vi "HEWH Flow Adjustment.vi"(0 "VISA session":refnum<visa-resource-name>="MW100", 1 "Configuration":T1=enum."SRK500,Station1,5GPM FR", 2 "Semiphore":T2, 5 "GPM Target(3)":dbl=3.0, 7 "GPM reading":dbl, 9 "Flow rate setting In":dbl=2.9360496277915633, 11 "Error In":errorcluster, 12 "Elapsed Time (sec)":dbl format="%.2f", 13 "Flow Adjust Time (3s)":dbl=3.0, 14 "K(0.1)":dbl=0.1) -> (4 "VISA session out":refnum<visa-resource-name>, 6 "Flow rate setting Out":dbl, 15 "Error Out":errorcluster)   [LabVIEW 2012]
uses:
  TestedFlowratesScenarios.ctl
  Intellifaucet/Intellfaucet Mode.ctl
panel:
  in  "ErrorPassBand(%)":dbl=0.05
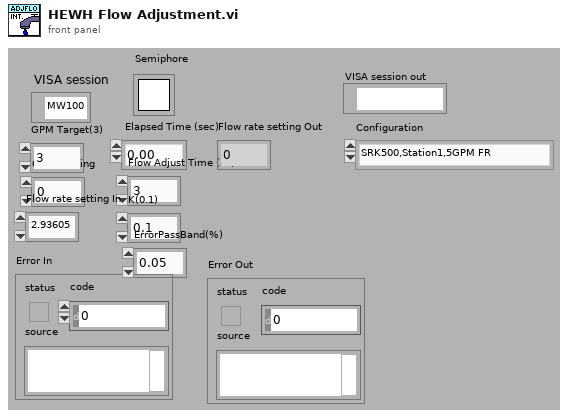
[diagram p1: front panel]
types:
  T1 = typedef "TestedFlowratesScenarios.ctl" = enum16{"DRK500,Station1", "DRK375,Lab", "SRK500,Station1,5GPM FR", "DRK375,STATION3,1/2\"HOSE", "DRK500,Station1,downspout", "DRK375,Station3,thruEcocute", "DRK375,Station3,purge", "Build2,2B,Purge", "Global, Purge", "Global, Tank"}
  T2 = typedef "Semaphore RefNum" = refnum<k1>
  T3 = typedef "Intellfaucet Mode.ctl" = enum16{"Adjust Temp", "Adjust Flow", "Start Flow", "Stop Flow"}
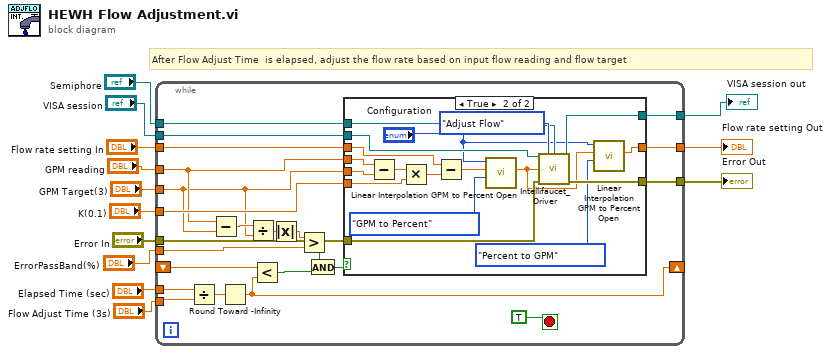
[diagram p0: block diagram]
diagram:
  # "After Flow Adjust Time  is elapsed, adjust the flow rate based on input flow reading and flow target"
  n1 = while {
    tunnel: "Elapsed Time (sec)" -> [w35]
    tunnel: "Flow Adjust Time (3s)" -> [w34]
    shift-right: [w24] -> _
    shift-left: _ -> [w25]
    tunnel: "VISA session" -> [w32]
    tunnel: "Semiphore" -> [w31]
    tunnel: "Error In" -> [w30]
    tunnel: [w29] -> w8
    tunnel: "GPM reading" -> [w20]
    tunnel: "GPM Target(3)" -> [w18]
    tunnel: "K(0.1)" -> [w28]
    tunnel: "Flow rate setting In" -> [w27]
    tunnel: [w26] -> w3
    tunnel: [w23] -> w2
    tunnel: "ErrorPassBand(%)" -> [w17]
    stop <- TRUE stop-if-true
    n2 = Divide(x=w35, y=w34) -> (x/y=w33:dbl)
    n3 = Subtract(x=w20, y=w18) -> (x-y=w19:dbl)
    n4 = Round Toward -Infinity(1:w33) -> (0:w24:dbl)
    n5 = Divide(x=w19, y=w18) -> (x/y=w14:dbl)
    n6 = Less?(x=w25, y=w24) -> (x < y?=w22:bool)
    n7 = Absolute Value(x=w14) -> (abs(x)=w15:dbl)
    n8 = Greater?(x=w15, y=w17) -> (0:w16:bool)
    n9 = And(x=w16, y=w22) -> (x .and. y?=w21:bool)
    n10 = case shown="True" w21 {
      tunnel: w32 -> [w37 w56]
      tunnel: w31 -> [_ w55]
      tunnel: w30 -> [w39 w54]
      tunnel: [w39 w53] -> w29
      tunnel: w28 -> [_ w51]
      tunnel: w18 -> [_ w50]
      tunnel: w20 -> [_ w49]
      tunnel: w27 -> [w38 w47]
      tunnel: [w38 w43] -> w26
      tunnel: [w37 w45] -> w23
      frame False {
      }
      frame True {
        n11 = Subtract(x=w49, y=w50) -> (x-y=w52:dbl)
        n12 = Multiply(x=w52, y=w51) -> (x*y=w48:dbl)
        n13 = Subtract(x=w47, y=w48) -> (x-y=w46:dbl)
        n14 = call "Linear Interpolation GPM to Percent Open.vi"("Interp Direction"=enum16{"GPM to Percent", "Percent to GPM"}."GPM to Percent", "Input (GPM,Percent)"=w46, "Configuration"="Configuration") -> ("Output (Percent,GPM)"=w42:dbl)  [unwired: 8 in]
        n15 = call "Intellifaucet_Driver.vi"("VISA session"=w56, "Mode"=Intellfaucet_Mode."Adjust Flow", "Semiphore"=w55, "Percent Flow"=w42, "Error In"=w54) -> ("VISA session out"=w45:refnum<visa-resource-name>, "Error Out"=w53:errorcluster)  [unwired: 9 in]
        n16 = call "Linear Interpolation GPM to Percent Open.vi"("Interp Direction"=enum16{"GPM to Percent", "Percent to GPM"}."Percent to GPM", "Input (GPM,Percent)"=w42, "Configuration"="Configuration") -> ("Output (Percent,GPM)"=w43:dbl)  [unwired: 8 in]
      }
    }
  }
  "Error Out" <- w8
  "Flow rate setting Out" <- w3
  "VISA session out" <- w2
